vi "ConfigureCamera.vi"(0 "Brightness::Mode":u32(ring)=2 items=["Manual"=2], 1 "Brightness::Value":u32 max=64 step=1, 2 "Contrast::Mode":u32(ring)=2 items=["Manual"=2], 3 "Contrast::Value":dbl min=0.0 max=1.0, 4 "Exposure::Mode":u32(ring)=1 items=["Auto"=1, "Manual"=2], 6 "Hue::Mode":u32(ring)=2 items=["Manual"=2], 7 "error in":errorcluster, 8 "Hue::Value":dbl min=-1.8 max=1.8, 9 "Saturation::Mode":u32(ring)=2 items=["Manual"=2], 10 "Saturation::Value":i64=64 min=0 max=100 step=1, 11 "Sharpness::Mode":u32(ring)=2 items=["Manual"=2], 12 "Sharpness::Value":i64=50 min=0 max=100 step=1, 13 "White Balance::Mode":u32(ring)=1 items=["Auto"=1, "Manual"=2], 16 "Session In":T2, 17 "Image In":T1, 19 "Exposure::Value":dbl caption="Hue::Value" min=-1.8 max=1.8, 21 "WhiteBalance::Value":dbl caption="Contrast::Value" min=0.0 max=1.0) -> (20 "Image Out":T1(plugin-control), 23 "Session Out":T2, 25 "Frame Rate":dbl, 26 "error out":errorcluster)   [LabVIEW 2020]
doc: "Creates, and edits acquisitions using the NI Vision Acquisition Express VI.\n\nThe NI Vision Acquisition Wizard is launched by placing the Express VI on the block diagram. Select an acquisition source and configure an acquisition using NI-IMAQ, NI-IMAQdx, or simulate an acquisition by reading an AVI or image files from a folder. After an acquisition is configured, select controls and indicators to be able to programmatically set in LabVIEW. Double-click the Vision Acquisition Express VI to edit the acquisition.\n\nNote: Any images created by the Express VI need to be disposed after use. Use the IMAQ Dispose.vi to cleanup the images output by the Express VI when they are no longer needed."
uses:
  <vilib>/userdefined/High Color/IMAQdx.ctl
  <vilib>/vision/Image Controls.llb/IMAQ Image.ctl
  <resource>/objmgr/imaqdx.rc
  <vilib>/vision/driver/NI_Vision_Acquisition_Software.lvlib
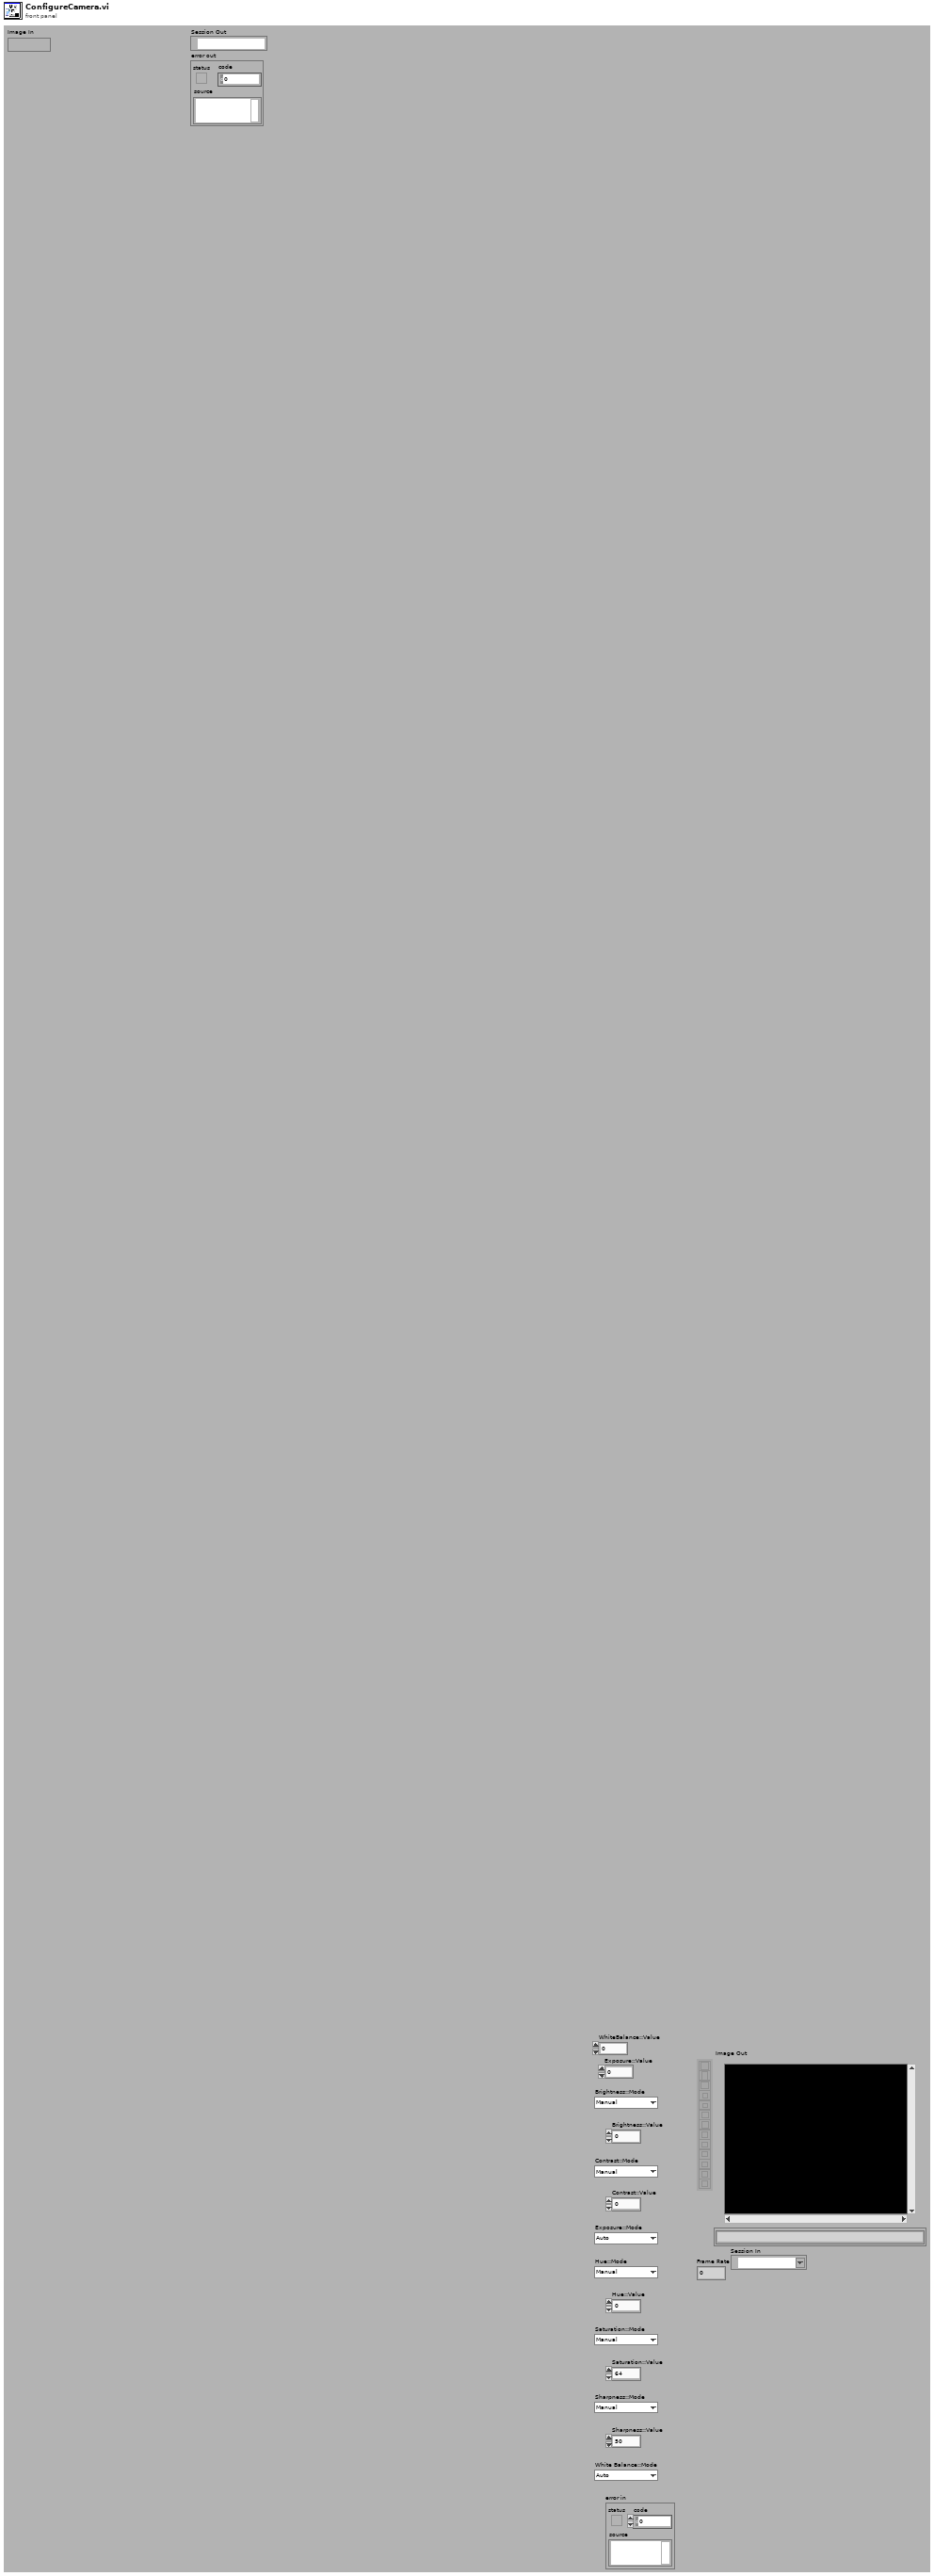
[diagram p1: front panel]
types:
  T1 = typedef "IMAQ Image.ctl" = refnum<image>
  T2 = typedef "IMAQdx.ctl" = refnum<k21>
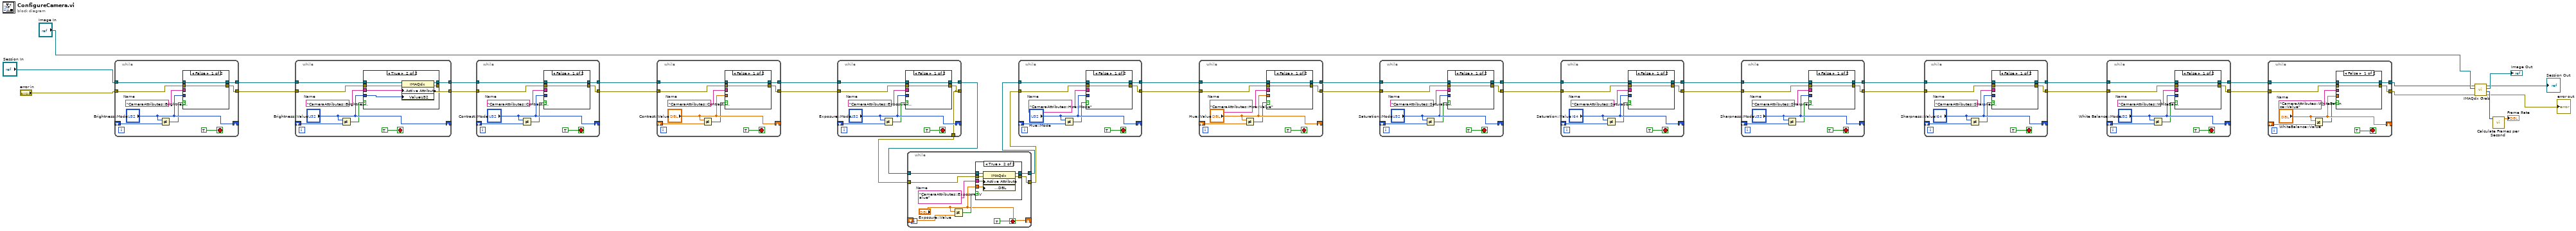
[diagram p0: block diagram]
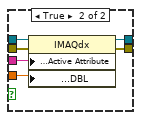
[diagram p3: hidden frame]
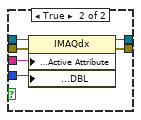
[diagram p4: hidden frame]
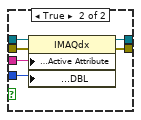
[diagram p5: hidden frame]
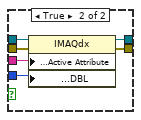
[diagram p6: hidden frame]
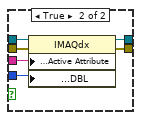
[diagram p7: hidden frame]
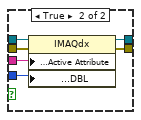
[diagram p8: hidden frame]
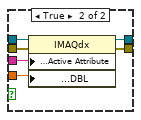
[diagram p9: hidden frame]
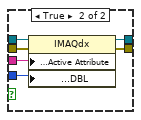
[diagram p10: hidden frame]
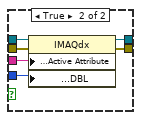
[diagram p11: hidden frame]
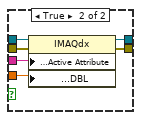
[diagram p12: hidden frame]
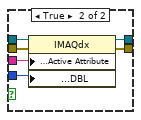
[diagram p13: hidden frame]
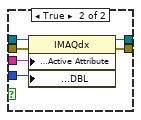
[diagram p15: hidden frame]
diagram:
  n1 = while {
    tunnel: "error in" -> [w45]
    tunnel: [w44] -> w35
    tunnel: "Session In" -> [w43]
    tunnel: [w42] -> w36
    shift-right: ["Brightness::Mode"] -> _
    shift-left: _ -> [w38]
    stop <- TRUE stop-if-true
    w41 = "CameraAttributes::Brightness::Mode"  # Name
    n2 = Not Equal?(x="Brightness::Mode", y=w38) -> (x != y?=w37:bool)
    n3 = case shown="False" w37 {
      tunnel: w45 -> [w46 w53]
      tunnel: [w47 w52] -> w44
      tunnel: w43 -> [w47 w51]
      tunnel: [w46 w50] -> w42
      tunnel: w41 -> [_ w49]
      tunnel: "Brightness::Mode" -> [_ w48]
      frame False {
      }
      frame True {
        n4 = property class="IMAQdx"(reference=w51, error in=w53, "Camera Attributes:Active Attribute"=w49, "Camera Attributes:Value:DBL"=w48) -> (reference out=w52:T2, error out=w50:errorcluster)
      }
    }
  }
  n5 = while {
    tunnel: w36 -> [w62]
    tunnel: [w61] -> w33
    tunnel: w35 -> [w60]
    tunnel: [w59] -> w34
    shift-right: ["Brightness::Value"] -> _
    shift-left: _ -> [w55]
    stop <- TRUE stop-if-true
    w58 = "CameraAttributes::Brightness::Value"  # Name
    n6 = Not Equal?(x="Brightness::Value", y=w55) -> (x != y?=w54:bool)
    n7 = case shown="True" w54 {
      tunnel: w62 -> [w63 w70]
      tunnel: [w64 w69] -> w61
      tunnel: w60 -> [w64 w68]
      tunnel: [w63 w67] -> w59
      tunnel: w58 -> [_ w66]
      tunnel: "Brightness::Value" -> [_ w65]
      frame False {
      }
      frame True {
        n8 = property class="IMAQdx"(reference=w68, error in=w70, "Camera Attributes:Active Attribute"=w66, "ValueU32"=w65) -> (reference out=w69:T2, error out=w67:errorcluster)
      }
    }
  }
  n9 = while {
    tunnel: w34 -> [w79]
    tunnel: [w78] -> w31
    tunnel: w33 -> [w77]
    tunnel: [w76] -> w32
    shift-right: ["Contrast::Mode"] -> _
    shift-left: _ -> [w72]
    stop <- TRUE stop-if-true
    w75 = "CameraAttributes::Contrast::Mode"  # Name
    n10 = Not Equal?(x="Contrast::Mode", y=w72) -> (x != y?=w71:bool)
    n11 = case shown="False" w71 {
      tunnel: w79 -> [w80 w87]
      tunnel: [w81 w86] -> w78
      tunnel: w77 -> [w81 w85]
      tunnel: [w80 w84] -> w76
      tunnel: w75 -> [_ w83]
      tunnel: "Contrast::Mode" -> [_ w82]
      frame False {
      }
      frame True {
        n12 = property class="IMAQdx"(reference=w85, error in=w87, "Camera Attributes:Active Attribute"=w83, "Camera Attributes:Value:DBL"=w82) -> (reference out=w86:T2, error out=w84:errorcluster)
      }
    }
  }
  n13 = while {
    tunnel: w32 -> [w96]
    tunnel: [w95] -> w29
    tunnel: w31 -> [w94]
    tunnel: [w93] -> w30
    shift-right: ["Contrast::Value"] -> _
    shift-left: _ -> [w89]
    stop <- TRUE stop-if-true
    w92 = "CameraAttributes::Contrast::Value"  # Name
    n14 = Not Equal?(x="Contrast::Value", y=w89) -> (x != y?=w88:bool)
    n15 = case shown="False" w88 {
      tunnel: w96 -> [w97 w104]
      tunnel: [w98 w103] -> w95
      tunnel: w94 -> [w98 w102]
      tunnel: [w97 w101] -> w93
      tunnel: w92 -> [_ w100]
      tunnel: "Contrast::Value" -> [_ w99]
      frame False {
      }
      frame True {
        n16 = property class="IMAQdx"(reference=w102, error in=w104, "Camera Attributes:Active Attribute"=w100, "Camera Attributes:Value:DBL"=w99) -> (reference out=w103:T2, error out=w101:errorcluster)
      }
    }
  }
  n17 = while {
    tunnel: w30 -> [w113]
    tunnel: [w112] -> w4
    tunnel: w29 -> [w111]
    tunnel: [w105] -> _
    shift-right: ["Exposure::Mode"] -> _
    shift-left: _ -> [w107]
    tunnel: [w105] -> w3
    stop <- TRUE stop-if-true
    w110 = "CameraAttributes::Exposure::Mode"  # Name
    n18 = Not Equal?(x="Exposure::Mode", y=w107) -> (x != y?=w106:bool)
    n19 = case shown="False" w106 {
      tunnel: w113 -> [w114 w121]
      tunnel: [w115 w120] -> w112
      tunnel: w111 -> [w115 w119]
      tunnel: [w114 w118] -> w105
      tunnel: w110 -> [_ w117]
      tunnel: "Exposure::Mode" -> [_ w116]
      frame False {
      }
      frame True {
        n20 = property class="IMAQdx"(reference=w119, error in=w121, "Camera Attributes:Active Attribute"=w117, "Camera Attributes:Value:DBL"=w116) -> (reference out=w120:T2, error out=w118:errorcluster)
      }
    }
  }
  n21 = while {
    tunnel: w3 -> [w130]
    tunnel: [w129] -> w2
    tunnel: w4 -> [w128]
    tunnel: [w127] -> w1
    shift-right: ["Exposure::Value"] -> _
    shift-left: _ -> [w124]
    stop <- TRUE stop-if-true
    w126 = "CameraAttributes::Exposure::Value"  # Name
    n22 = Not Equal?(x="Exposure::Value", y=w124) -> (x != y?=w123:bool)
    n23 = case shown="True" w123 {
      tunnel: w130 -> [w131 w138]
      tunnel: [w132 w137] -> w129
      tunnel: w128 -> [w132 w136]
      tunnel: [w131 w135] -> w127
      tunnel: w126 -> [_ w134]
      tunnel: "Exposure::Value" -> [_ w133]
      frame False {
      }
      frame True {
        n24 = property class="IMAQdx"(reference=w136, error in=w138, "Camera Attributes:Active Attribute"=w134, "Camera Attributes:Value:DBL"=w133) -> (reference out=w137:T2, error out=w135:errorcluster)
      }
    }
  }
  n25 = while {
    tunnel: w1 -> [w147]
    tunnel: [w146] -> w27
    tunnel: w2 -> [w145]
    tunnel: [w144] -> w28
    shift-right: ["Hue::Mode"] -> _
    shift-left: _ -> [w140]
    stop <- TRUE stop-if-true
    w143 = "CameraAttributes::Hue::Mode"  # Name
    n26 = Not Equal?(x="Hue::Mode", y=w140) -> (x != y?=w139:bool)
    n27 = case shown="False" w139 {
      tunnel: w147 -> [w148 w155]
      tunnel: [w149 w154] -> w146
      tunnel: w145 -> [w149 w153]
      tunnel: [w148 w152] -> w144
      tunnel: w143 -> [_ w151]
      tunnel: "Hue::Mode" -> [_ w150]
      frame False {
      }
      frame True {
        n28 = property class="IMAQdx"(reference=w153, error in=w155, "Camera Attributes:Active Attribute"=w151, "Camera Attributes:Value:DBL"=w150) -> (reference out=w154:T2, error out=w152:errorcluster)
      }
    }
  }
  n29 = while {
    tunnel: w28 -> [w164]
    tunnel: [w163] -> w25
    tunnel: w27 -> [w162]
    tunnel: [w161] -> w26
    shift-right: ["Hue::Value"] -> _
    shift-left: _ -> [w157]
    stop <- TRUE stop-if-true
    w160 = "CameraAttributes::Hue::Value"  # Name
    n30 = Not Equal?(x="Hue::Value", y=w157) -> (x != y?=w156:bool)
    n31 = case shown="False" w156 {
      tunnel: w164 -> [w165 w172]
      tunnel: [w166 w171] -> w163
      tunnel: w162 -> [w166 w170]
      tunnel: [w165 w169] -> w161
      tunnel: w160 -> [_ w168]
      tunnel: "Hue::Value" -> [_ w167]
      frame False {
      }
      frame True {
        n32 = property class="IMAQdx"(reference=w170, error in=w172, "Camera Attributes:Active Attribute"=w168, "Camera Attributes:Value:DBL"=w167) -> (reference out=w171:T2, error out=w169:errorcluster)
      }
    }
  }
  n33 = while {
    tunnel: w26 -> [w181]
    tunnel: [w180] -> w23
    tunnel: w25 -> [w179]
    tunnel: [w178] -> w24
    shift-right: ["Saturation::Mode"] -> _
    shift-left: _ -> [w174]
    stop <- TRUE stop-if-true
    w177 = "CameraAttributes::Saturation::Mode"  # Name
    n34 = Not Equal?(x="Saturation::Mode", y=w174) -> (x != y?=w173:bool)
    n35 = case shown="False" w173 {
      tunnel: w181 -> [w182 w189]
      tunnel: [w183 w188] -> w180
      tunnel: w179 -> [w183 w187]
      tunnel: [w182 w186] -> w178
      tunnel: w177 -> [_ w185]
      tunnel: "Saturation::Mode" -> [_ w184]
      frame False {
      }
      frame True {
        n36 = property class="IMAQdx"(reference=w187, error in=w189, "Camera Attributes:Active Attribute"=w185, "Camera Attributes:Value:DBL"=w184) -> (reference out=w188:T2, error out=w186:errorcluster)
      }
    }
  }
  n37 = while {
    tunnel: w24 -> [w198]
    tunnel: [w197] -> w21
    tunnel: w23 -> [w196]
    tunnel: [w195] -> w22
    shift-right: ["Saturation::Value"] -> _
    shift-left: _ -> [w191]
    stop <- TRUE stop-if-true
    w194 = "CameraAttributes::Saturation::Value"  # Name
    n38 = Not Equal?(x="Saturation::Value", y=w191) -> (x != y?=w190:bool)
    n39 = case shown="False" w190 {
      tunnel: w198 -> [w199 w206]
      tunnel: [w200 w205] -> w197
      tunnel: w196 -> [w200 w204]
      tunnel: [w199 w203] -> w195
      tunnel: w194 -> [_ w202]
      tunnel: "Saturation::Value" -> [_ w201]
      frame False {
      }
      frame True {
        n40 = property class="IMAQdx"(reference=w204, error in=w206, "Camera Attributes:Active Attribute"=w202, "Camera Attributes:Value:DBL"=w201) -> (reference out=w205:T2, error out=w203:errorcluster)
      }
    }
  }
  n41 = while {
    tunnel: w22 -> [w215]
    tunnel: [w214] -> w19
    tunnel: w21 -> [w213]
    tunnel: [w212] -> w20
    shift-right: ["Sharpness::Mode"] -> _
    shift-left: _ -> [w208]
    stop <- TRUE stop-if-true
    w211 = "CameraAttributes::Sharpness::Mode"  # Name
    n42 = Not Equal?(x="Sharpness::Mode", y=w208) -> (x != y?=w207:bool)
    n43 = case shown="False" w207 {
      tunnel: w215 -> [w216 w223]
      tunnel: [w217 w222] -> w214
      tunnel: w213 -> [w217 w221]
      tunnel: [w216 w220] -> w212
      tunnel: w211 -> [_ w219]
      tunnel: "Sharpness::Mode" -> [_ w218]
      frame False {
      }
      frame True {
        n44 = property class="IMAQdx"(reference=w221, error in=w223, "Camera Attributes:Active Attribute"=w219, "Camera Attributes:Value:DBL"=w218) -> (reference out=w222:T2, error out=w220:errorcluster)
      }
    }
  }
  n45 = while {
    tunnel: w20 -> [w232]
    tunnel: [w231] -> w17
    tunnel: w19 -> [w230]
    tunnel: [w229] -> w18
    shift-right: ["Sharpness::Value"] -> _
    shift-left: _ -> [w225]
    stop <- TRUE stop-if-true
    w228 = "CameraAttributes::Sharpness::Value"  # Name
    n46 = Not Equal?(x="Sharpness::Value", y=w225) -> (x != y?=w224:bool)
    n47 = case shown="False" w224 {
      tunnel: w232 -> [w233 w240]
      tunnel: [w234 w239] -> w231
      tunnel: w230 -> [w234 w238]
      tunnel: [w233 w237] -> w229
      tunnel: w228 -> [_ w236]
      tunnel: "Sharpness::Value" -> [_ w235]
      frame False {
      }
      frame True {
        n48 = property class="IMAQdx"(reference=w238, error in=w240, "Camera Attributes:Active Attribute"=w236, "Camera Attributes:Value:DBL"=w235) -> (reference out=w239:T2, error out=w237:errorcluster)
      }
    }
  }
  n49 = while {
    tunnel: w18 -> [w249]
    tunnel: [w248] -> w8
    tunnel: w17 -> [w247]
    tunnel: [w246] -> w7
    shift-right: ["White Balance::Mode"] -> _
    shift-left: _ -> [w242]
    stop <- TRUE stop-if-true
    w245 = "CameraAttributes::WhiteBalance::Mode"  # Name
    n50 = Not Equal?(x="White Balance::Mode", y=w242) -> (x != y?=w241:bool)
    n51 = case shown="False" w241 {
      tunnel: w249 -> [w250 w257]
      tunnel: [w251 w256] -> w248
      tunnel: w247 -> [w251 w255]
      tunnel: [w250 w254] -> w246
      tunnel: w245 -> [_ w253]
      tunnel: "White Balance::Mode" -> [_ w252]
      frame False {
      }
      frame True {
        n52 = property class="IMAQdx"(reference=w255, error in=w257, "Camera Attributes:Active Attribute"=w253, "Camera Attributes:Value:DBL"=w252) -> (reference out=w256:T2, error out=w254:errorcluster)
      }
    }
  }
  n53 = while {
    tunnel: w7 -> [w266]
    tunnel: [w265] -> w6
    tunnel: w8 -> [w264]
    tunnel: [w263] -> w5
    shift-right: ["WhiteBalance::Value"] -> _
    shift-left: _ -> [w260]
    stop <- TRUE stop-if-true
    w258 = "CameraAttributes::WhiteBalance::Value"  # Name
    n54 = Not Equal?(x="WhiteBalance::Value", y=w260) -> (x != y?=w259:bool)
    n55 = case shown="False" w259 {
      tunnel: w266 -> [w267 w274]
      tunnel: [w268 w273] -> w265
      tunnel: w264 -> [w268 w272]
      tunnel: [w267 w271] -> w263
      tunnel: w258 -> [_ w270]
      tunnel: "WhiteBalance::Value" -> [_ w269]
      frame False {
      }
      frame True {
        n56 = property class="IMAQdx"(reference=w272, error in=w274, "Camera Attributes:Active Attribute"=w270, "Camera Attributes:Value:DBL"=w269) -> (reference out=w273:T2, error out=w271:errorcluster)
      }
    }
  }
  n57 = call <vilib>:"IMAQdx Grab.vi"("error in"=w5, "Image In"="Image In", "Session In"=w6) -> ("error out"=→"error out":errorcluster, "Buffer Number Out"=w15:u32, "Image Out"=→"Image Out":T1, "Session Out"=→"Session Out":T2)  [unwired: 1 in, 4 out]
  n58 = call <vilib>:"Calculate Frames per Second.vi"("Buffer Number"=w15) -> ("Acquired Frames/s"=→"Frame Rate":dbl)  [unwired: 2 in, 8 out]
